vi "DriveToXY.vi"(1 "Drive Margin":dbl=12.0, 2 "Steer Margin":dbl=10.0, 5 "X Target":dbl, 7 "Y Target":dbl, 9 "Speed":dbl, 11 "error in":errorcluster, 12 "Start time":u32, 13 "Timeout (ms)":u32=2000) -> (4 "RobotDriveDevRef Out":T1={"DevStatus"={"status"=FALSE, "code"=0, "source"=""}, "Motors[]"=[], "Square Inputs"=FALSE, "Max Output"=1.0, "Isochronous"=FALSE}, 6 "At Target":bool, 8 "Timeout?":bool, 15 "error out":errorcluster)   [LabVIEW 2013]
uses:
  <vilib>/Rock Robotics/WPI/RobotDrive/WPI_RobotDriveDevRef.ctl
  <vilib>/Rock Robotics/WPI/MotorControl/WPI_MotorControlDeviceRef.ctl
  <vilib>/Rock Robotics/SystemInterfaces/Typedef/FPGA_TypedefDigitalModule.ctl
  <vilib>/Rock Robotics/SystemInterfaces/DIO/FPGA_DIOPWMChannel.ctl
  <vilib>/Rock Robotics/WPI/PWM/WPI_PWMDeadband.ctl
  <vilib>/Rock Robotics/WPI/CAN/Jaguar/SubVIs/WPI_CANJaguar_ControlMode.ctl
  <vilib>/Rock Robotics/WPI/PWM/WPI_PWMTransform_ConPane.ctl
  Robot Global Data.vi
  <vilib>/Rock Robotics/WPI/RobotDrive/WPI_RobotDriveGetSetRefNum.vi
  <vilib>/addons/control/pid/NI_PID_pid.lvlib
panel:
  out "Waveform Chart":dbl(graph)
  in  "Drive PID gains":T9={"proportional gain (Kc)"=0.12, "integral time (Ti, min)"=0.0, "derivative time (Td, min)"=0.0} {"derivative time (Td, min)" format="%.3f"; "integral time (Ti, min)" format="%.3f"; "proportional gain (Kc)" format="%.3f"}
  in  "Steer PID gains":T9={"proportional gain (Kc)"=0.05, "integral time (Ti, min)"=0.01, "derivative time (Td, min)"=0.002} {"derivative time (Td, min)" format="%#.7g"; "integral time (Ti, min)" format="%#.6g"; "proportional gain (Kc)" format="%#.6g"}
  in  "Steering Saturation":dbl=1.0
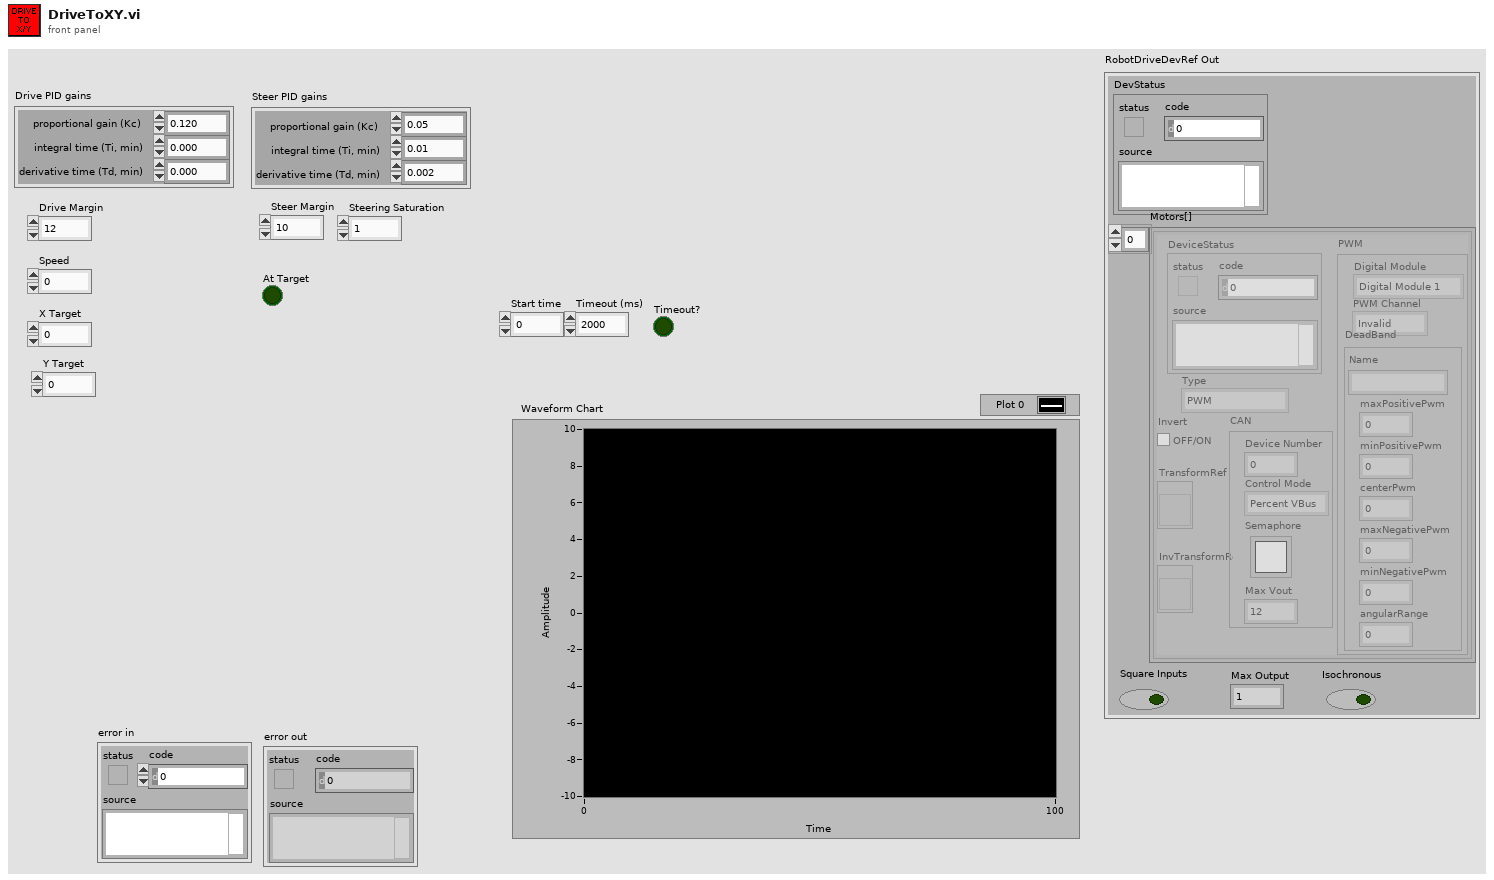
[diagram p1: front panel]
types:
  T1 = typedef "WPI_RobotDriveDevRef.ctl" = cluster{"DevStatus":errorcluster, "Motors[]":T2[], "Square Inputs":bool, "Max Output":dbl, "Isochronous":bool}
  T2 = typedef "WPI_MotorControlDeviceRef.ctl" = cluster{"DeviceStatus":errorcluster, "Type":enum16{"PWM", "CAN"}, "PWM":cluster{"Digital Module":T3, "PWM Channel":T4, "DeadBand":T5}, "CAN":cluster{"Device Number":u8, "Control Mode":T6, "Semaphore":T7, "Max Vout":dbl}, "Invert":bool, "TransformRef":T8, "InvTransformRef":T8}
  T3 = typedef "FPGA_TypedefDigitalModule.ctl" = enum16{"Digital Module 1", "Digital Module 2"}
  T4 = typedef "FPGA_DIOPWMChannel.ctl" = enum8{"PWM 1", "PWM 2", "PWM 3", "PWM 4", "PWM 5", "PWM 6", "PWM 7", "PWM 8", "PWM 9", "PWM 10", "Invalid"}
  T5 = typedef "WPI_PWMDeadband.ctl" = cluster{"Name":string, "maxPositivePwm":i32, "minPositivePwm":i32, "centerPwm":i32, "maxNegativePwm":i32, "minNegativePwm":i32, "angularRange":u16}
  T6 = typedef "WPI_CANJaguar_ControlMode.ctl" = enum8{"Percent VBus", "Current", "Speed", "Position", "Voltage"}
  T7 = typedef "Semaphore RefNum" = refnum<k1>
  T8 = typedef "WPI_PWMTransform_ConPane.ctl" = refnum<vi>
  T9 = cluster{"proportional gain (Kc)":dbl, "integral time (Ti, min)":dbl, "derivative time (Td, min)":dbl}
  T10 = typedef "Position Typedef.ctl" = cluster{"X":dbl, "Y":dbl, "Heading":dbl}
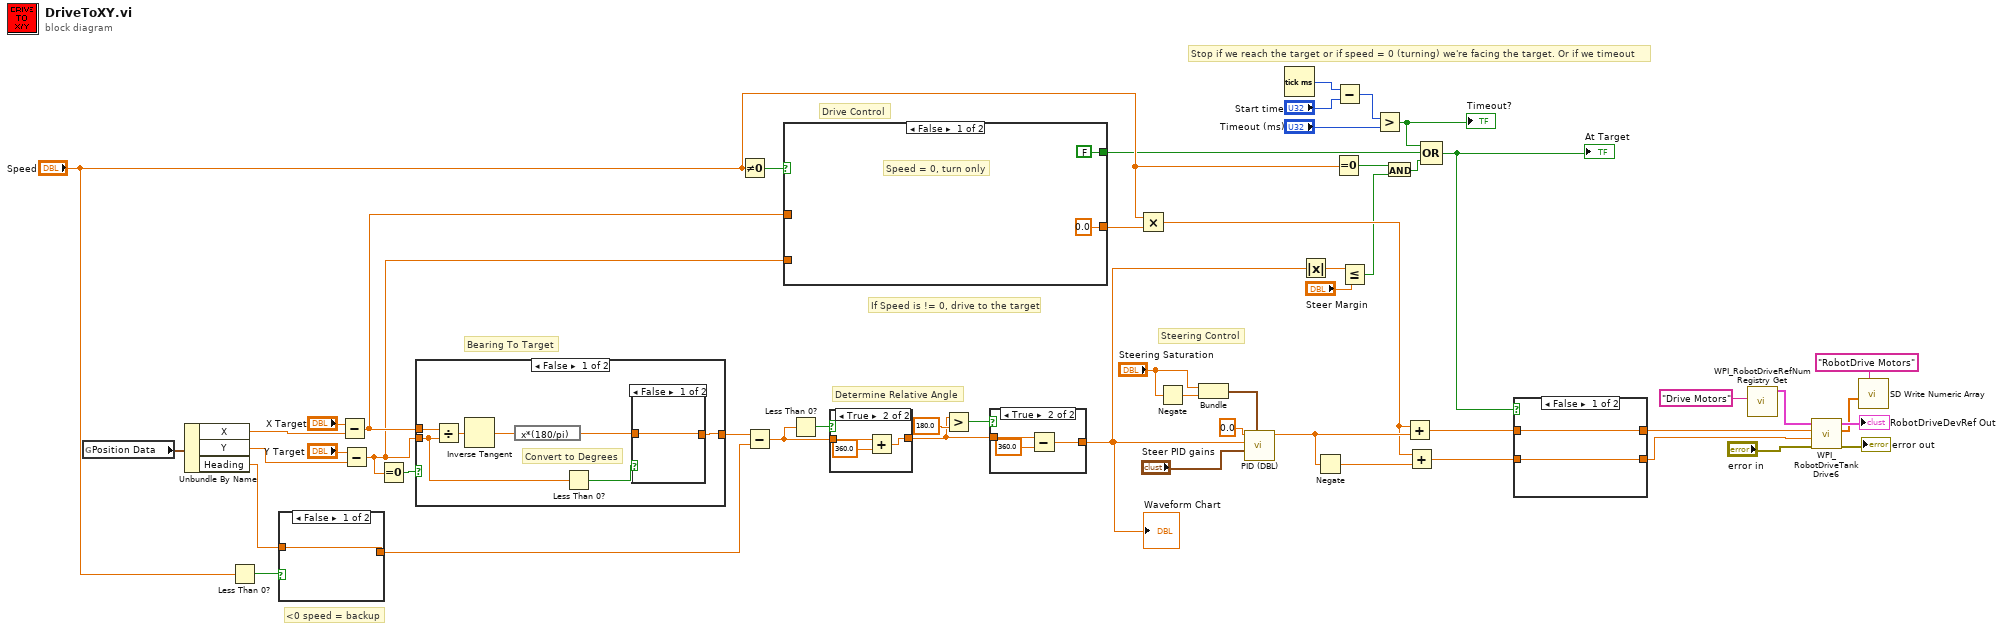
[diagram p0: block diagram]
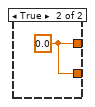
[diagram p2: hidden frame]
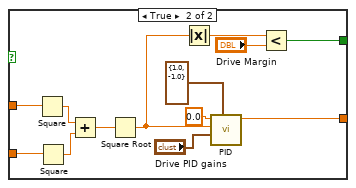
[diagram p3: hidden frame]
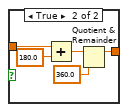
[diagram p6: hidden frame]
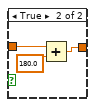
[diagram p7: hidden frame]
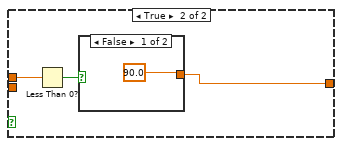
[diagram p8: hidden frame]
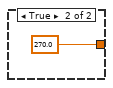
[diagram p9: hidden frame]
diagram:
  # "Stop if we reach the target or if speed = 0 (turning) we're facing the target. Or if we timeout"
  # "Drive Control"
  # "If Speed is != 0, drive to the target"
  # "Steering Control"
  # "Determine Relative Angle"
  # "Bearing To Target"
  # "<0 speed = backup"
  n1 = global read "Robot Global Data.vi" "Position Data"() -> (w52:T10)
  n2 = Unbundle By Name(w52) -> ("X"=w34:dbl, "Y"=w33:dbl, "Heading"=w48:dbl)
  n3 = Less Than 0?(x="Speed") -> (x < 0?=w45:bool)
  n4 = case shown="False" w45 {
    tunnel: w48 -> [w53 w55]
    tunnel: [w53 w54] -> w46
    frame False {
    }
    frame True {
      n5 = Add(x=w55, y=180.0) -> (x+y=w57:dbl)
      n6 = Quotient & Remainder(x=w57, y=360.0) -> (x-y*floor(x/y)=w54:dbl)  [unwired: 1 out]
    }
  }
  n7 = Subtract(x="X Target", y=w34) -> (x-y=w32:dbl)
  n8 = Subtract(x="Y Target", y=w33) -> (x-y=w31:dbl)
  n9 = Equal To 0?(x=w31) -> (x = 0?=w49:bool)
  n10 = case shown="False" w49 {
    tunnel: w32 -> [w65 w71]
    tunnel: [w60 w70] -> w47
    tunnel: w31 -> [w62 _]
    frame False {
      # "Convert to Degrees"
      n11 = Divide(x=w65, y=w62) -> (x/y=w63:dbl)
      n12 = Inverse Tangent(1:w63) -> (0:w64:dbl)
      n13 = expression code="x*(180/pi)"(w64) -> (w59:dbl)
      n14 = Less Than 0?(x=w62) -> (x < 0?=w61:bool)
      n15 = case shown="False" w61 {
        tunnel: [w66 w69] -> w60
        tunnel: w59 -> [w66 w68]
        frame False {
        }
        frame True {
          n16 = Add(x=w68, y=180.0) -> (x+y=w69:dbl)
        }
      }
    }
    frame True {
      n17 = Less Than 0?(x=w71) -> (x < 0?=w72:bool)
      n18 = case shown="False" w72 {
        tunnel: [90.0 ("y") 270.0 ("y")] -> w70
        frame False {
        }
        frame True {
        }
      }
    }
  }
  n19 = Not Equal To 0?(x="Speed") -> (x != 0?=w28:bool)
  n20 = Subtract(x=w47, y=w46) -> (x-y=w40:dbl)
  n21 = case shown="False" w28 {
    tunnel: w32 -> [_ w80]
    tunnel: w31 -> [_ w79]
    tunnel: [FALSE w78] -> w22
    tunnel: [0.0 ("output") w77] -> w27
    frame False {
      # "Speed = 0, turn only"
    }
    frame True {
      n22 = Square(x=w80) -> (x^2=w87:dbl)
      n23 = Square(x=w79) -> (x^2=w86:dbl)
      n24 = Add(x=w87, y=w86) -> (x+y=w85:dbl)
      n25 = Square Root(x=w85) -> (sqrt(x)=w82:dbl)
      n26 = Absolute Value(x=w82) -> (abs(x)=w84:dbl)
      n27 = call-poly <vilib>:"PID.vi"("output range"=cluster{"output high":dbl, "output low":dbl} {"output high"=1.0, "output low"=-1.0}, "PID gains"="Drive PID gains", "process variable"=w82, "setpoint"=0.0 ("y")) -> ("output"=w77:dbl)  [unwired: 2 in, 5 out]
      n28 = Less?(x=w84, y="Drive Margin") -> (x < y?=w78:bool)
    }
  }
  n29 = Less Than 0?(x=w40) -> (x < 0?=w42:bool)
  n30 = case shown="True" w42 {
    tunnel: w40 -> [w90 w92]
    tunnel: [w90 w91] -> w41
    frame False {
    }
    frame True {
      n31 = Add(x=w92, y=360.0) -> (x+y=w91:dbl)
    }
  }
  n32 = Greater?(x=w41, y=180.0) -> (0:w43:bool)
  n33 = case shown="True" w43 {
    tunnel: w41 -> [w94 w97]
    tunnel: [w94 w96] -> w1
    frame False {
    }
    frame True {
      n34 = Subtract(x=w97, y=360.0) -> (x-y=w96:dbl)
    }
  }
  "Waveform Chart" <- w1
  n35 = Multiply(x="Speed", y=w27) -> (x*y=w24:dbl)
  n36 = Negate(x="Steering Saturation") -> (-x=w38:dbl)
  n37 = Bundle("Steering Saturation"="Steering Saturation", w38) -> (w37:cluster{"Steering Saturation":dbl, dbl})  [unwired: 1 out]
  n38 = call <vilib>:"PID (DBL).vi"("output range"=w37, "PID gains"="Steer PID gains", "process variable"=w1, "setpoint"=0.0) -> ("output"=w26:dbl)  [unwired: 2 in, 5 out]
  n39 = Tick Count (ms)() -> (millisecond timer value=w11:u32)
  n40 = Absolute Value(x=w1) -> (abs(x)=w30:dbl)
  n41 = Negate(x=w26) -> (-x=w25:dbl)
  n42 = Equal To 0?(x="Speed") -> (x = 0?=w20:bool)
  n43 = Subtract(x=w11, y="Start time") -> (x-y=w10:u32)
  n44 = Less Or Equal?(x=w30, y="Steer Margin") -> (x <= y?=w19:bool)
  n45 = Greater?(x=w10, y="Timeout (ms)") -> (0:w7:bool)
  "Timeout?" <- w7
  n46 = And(x=w20, y=w19) -> (x .and. y?=w21:bool)
  n47 = Add(x=w24, y=w26) -> (x+y=w5:dbl)
  n48 = Add(x=w24, y=w25) -> (x+y=w4:dbl)
  n49 = Compound Arithmetic op=OR(w7, w22, w21) -> (w6:bool)
  "At Target" <- w6
  n50 = case shown="False" w6 {
    tunnel: w5 -> [w99 _]
    tunnel: w4 -> [w98 _]
    tunnel: [w99 w100] -> w3
    tunnel: [w98 w100] -> w2
    frame False {
    }
    frame True {
      w100 = 0.0
    }
  }
  n51 = call <vilib>:"WPI_RobotDriveRefNum Registry Get.vi"("refnum name"="Drive Motors") -> ("RobotDriveDevRef"=w16:T1)  [unwired: 1 in, 9 out]
  n52 = call "WPI_RobotDriveTankDrive6.vi"("error in (no error)"="error in", "Right axis value"=w2, "Left axis value"=w3, "RobotDriveDevRef"=w16) -> ("error out"=→"error out":errorcluster, "Motor Values"=w12:dbl[], "RobotDriveDevRef"=→"RobotDriveDevRef Out":T1)  [unwired: 5 in]
  n53 = call <vilib>:"SD Write Numeric Array.vi"("Numeric Array"=w12, "Name"="RobotDrive Motors") -> ()  [unwired: 8 in, 2 out]
